vi "Waveform History Builder.vi"(10 "Waveform history (10 s)":dbl=10.0 format="%#_13g", 11 "Data Read":cluster{waveform(dbl)[], string[]}) -> (0 "Min Time":timestamp, 1 "Max Time":timestamp, 2 "Waveforms":waveform(dbl)[](array[waveform]), 3 "Channel Names":string[](array[string]))   [LabVIEW 2024]
uses:
  <vilib>/Waveform/WDTOps.llb/WDT Append Waveforms DBL.vi
  <vilib>/Waveform/WDTOps.llb/WDT Get Waveform Subset DBL.vi
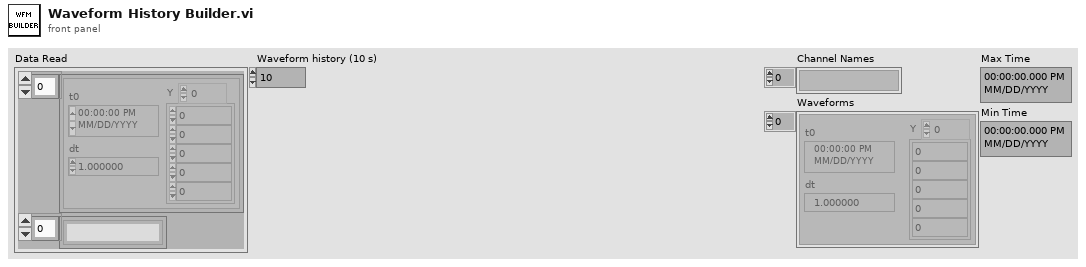
[diagram p1: front panel]
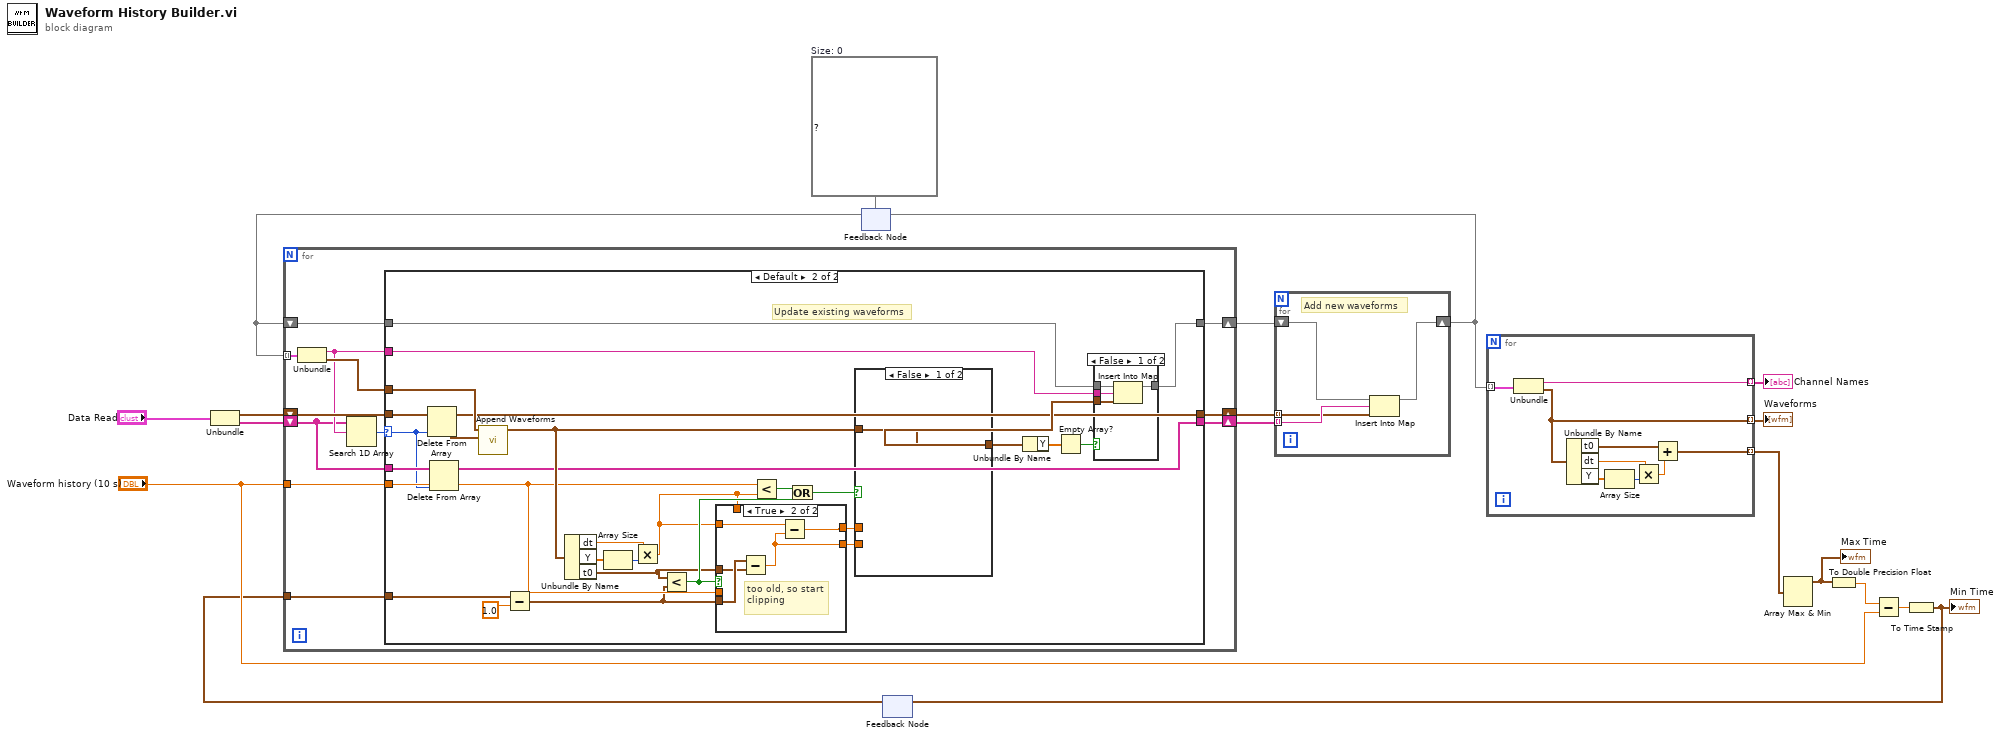
[diagram p0: block diagram]
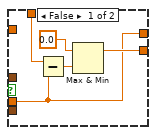
[diagram p3: hidden frame]
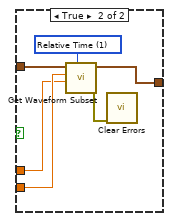
[diagram p4: hidden frame]
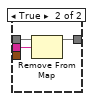
[diagram p5: hidden frame]
diagram:
  w16 = map{string, waveform(dbl)} {}  # Size: 0
  n1 = Unbundle("Data Read") -> (w9:waveform(dbl)[], w17:string[])
  n2 = feedback #1(w16) -> (w8:map{string, waveform(dbl)})
  n3 = feedback #2() -> (w2:timestamp)  [unwired: 1 in]
  n4 = for {
    tunnel: "Waveform history (10 s)" -> [w21]
    tunnel: w8 -> [w30] mode=indexing
    shift-right: [w25] -> w5
    shift-left: w8 -> [w27]
    shift-right: [w22] -> w7
    shift-left: w9 -> [w29]
    shift-right: [w23] -> w6
    shift-left: w17 -> [w24]
    tunnel: w2 -> [w20]
    n5 = Unbundle(w30) -> (w26:string, "Waveform"=w28:waveform(dbl))
    n6 = Search 1D Array(1D array=w24, element=w26) -> (index of element=w19:i32)  [unwired: 1 in]
    n7 = case shown="Default" w19 {
      selector: w19 -> [_ w35]
      tunnel: w29 -> [w32 w61]
      tunnel: w28 -> [_ w60]
      tunnel: w27 -> [w33 w51]
      tunnel: w26 -> [_ w50]
      tunnel: [w33 w49] -> w25
      tunnel: w24 -> [w31 w48]
      tunnel: [w31 w47] -> w23
      tunnel: [w32 w46] -> w22
      tunnel: w21 -> [_ w45]
      tunnel: w20 -> [_ w39]
      frame -1 {
      }
      frame Default {
        # "Update existing waveforms"
        n8 = Delete From Array(array=w61, index=w35) -> (deleted portion=w34:waveform(dbl), array with subset deleted=w46:waveform(dbl)[])  [unwired: 1 in]
        n9 = Delete From Array(array=w48, index=w35) -> (array with subset deleted=w47:string[])  [unwired: 1 in, 1 out]
        n10 = call-poly <vilib>:"Append Waveforms.vi"("waveform B"=w34, "waveform A"=w60) -> ("waveform out"=w56:waveform(dbl))  [unwired: 8 in, 1 out]
        n11 = Subtract(x=w39, y=1.0) -> (x-y=w38:timestamp)
        n12 = Unbundle By Name(w56) -> ("dt"=w53:dbl, "Y"=w55:dbl[], "t0"=w37:timestamp)
        n13 = Array Size(array=w55) -> (size(s)=w54:i32)
        n14 = Multiply(x=w53, y=w54) -> (x*y=w36:dbl)
        n15 = Less?(x=w37, y=w38) -> (x < y?=w41:bool)
        n16 = case shown="True" w41 {
          tunnel: [w64 w68] -> w52
          tunnel: w45 -> [w62 _]
          tunnel: w36 -> [w63 _]
          tunnel: [w62 w67] -> w40
          tunnel: w38 -> [_ w71]
          tunnel: w37 -> [_ w70]
          tunnel: w36 -> [_ w69]
          frame False {
            n17 = Subtract(x=w63, y=w62) -> (x-y=w66:dbl)
            n18 = Max & Min(x=0.0 ("lower limit"), y=w66) -> (max(x,y)=w64:dbl)  [unwired: 1 out]
          }
          frame True {
            # "too old, so start clipping"
            n19 = Subtract(x=w71, y=w70) -> (x-y=w68:dbl)
            n20 = Subtract(x=w69, y=w68) -> (x-y=w67:dbl)
          }
        }
        n21 = Less?(x=w45, y=w36) -> (x < y?=w44:bool)
        n22 = Or(x=w44, y=w41) -> (x .or. y?=w43:bool)
        n23 = case shown="False" w43 {
          tunnel: [w72 w77] -> w58
          tunnel: w56 -> [w72 w76]
          tunnel: w52 -> [_ w75]
          tunnel: w40 -> [_ w74]
          frame False {
          }
          frame True {
            w78 = u16 1 items=["Samples", "Relative Time"] ("start/duration format")
            n24 = call-poly <vilib>:"Get Waveform Subset.vi"("start/duration format"=w78, "duration"=w74, "start samples/time"=w75, "waveform in"=w76) -> ("error out"=w73:errorcluster, "waveform out"=w77:waveform(dbl))  [unwired: 2 in, 2 out]
            n25 = call <vilib>:"Clear Errors.vi"("error in (no error)"=w73) -> ()  [unwired: 5 in, 2 out]
          }
        }
        n26 = Unbundle By Name(w58) -> ("Y"=w59:dbl[])
        n27 = Empty Array?(array=w59) -> (empty?=w57:bool)
        n28 = case shown="False" w57 {
          tunnel: w51 -> [w79 w85]
          tunnel: w50 -> [w82 w84]
          tunnel: [w80 w83] -> w49
          tunnel: w58 -> [w81 _]
          frame False {
            n29 = Insert Into Map(map in=w79, key=w82, value=w81) -> (map out=w80:map{string, waveform(dbl)})  [unwired: 2 out]
          }
          frame True {
            n30 = Remove From Map(10:w84, 11:w85) -> (3:w83:map{string, waveform(dbl)})  [unwired: 2 out]
          }
        }
      }
    }
  }
  n31 = for {
    tunnel: w7 -> [w87] mode=indexing
    tunnel: w6 -> [w88] mode=indexing
    shift-right: [w86] -> w4
    shift-left: w5 -> [w89]
    # "Add new waveforms"
    n32 = Insert Into Map(map in=w89, key=w88, value=w87) -> (map out=w86:map{string, waveform(dbl)})  [unwired: 2 out]
  }
  n33 = feedback-in #1(w4) -> ()
  n34 = for {
    tunnel: w4 -> [w98] mode=indexing
    tunnel: [w97] -> w15 mode=indexing
    tunnel: [w91] -> w14 mode=indexing
    tunnel: [w90] -> w10 mode=indexing
    n35 = Unbundle(w98) -> (w97:string, "Waveform"=w91:waveform(dbl))
    n36 = Unbundle By Name(w91) -> ("t0"=w93:timestamp, "dt"=w94:dbl, "Y"=w96:dbl[])
    n37 = Array Size(array=w96) -> (size(s)=w95:i32)
    n38 = Multiply(x=w94, y=w95) -> (x*y=w92:dbl)
    n39 = Add(x=w93, y=w92) -> (x+y=w90:timestamp)
  }
  "Channel Names" <- w15
  "Waveforms" <- w14
  n40 = Array Max & Min(array=w10) -> (max value=w3:timestamp)  [unwired: 3 out]
  "Max Time" <- w3
  n41 = To Double Precision Float(number=w3) -> (double precision float=w13:dbl)
  n42 = Subtract(x=w13, y="Waveform history (10 s)") -> (x-y=w11:dbl)
  n43 = To Time Stamp(1:w11) -> (0:w1:timestamp)
  "Min Time" <- w1
  n44 = feedback-in #2(w1) -> ()
